vi "Data.vi"(11 "Last Ack Msg in":refnum<class "Last Ack Msg.lvclass">) -> (2 "Actor":refnum<class "Actor.lvclass">)   [LabVIEW 2021, in "Last Ack.lvlib" / "Last Ack Msg.lvclass"]
uses:
  Last Ack Msg.lvclass
  jettl/Actor/Actor.lvclass
  Last Ack Msg.lvclass/Last Ack Msg.ctl
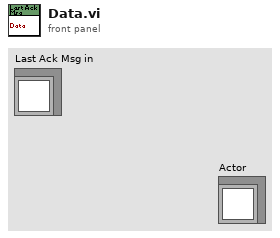
[diagram p1: front panel]
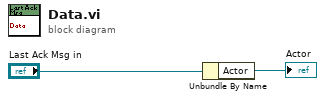
[diagram p0: block diagram]
diagram:
  n1 = Unbundle By Name("Last Ack Msg in") -> ("Actor"=→"Actor":refnum<class "Actor.lvclass">)
